vi "Get Message.vi"() -> (3 "message":string)   [LabVIEW 2014]
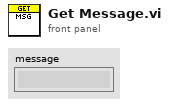
[diagram p1: front panel]
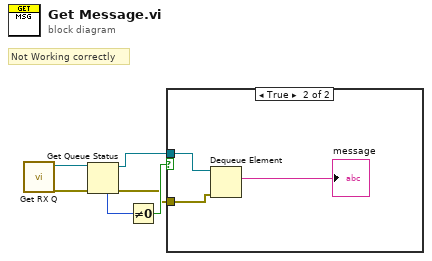
[diagram p0: block diagram]
diagram:
  # "Not Working correctly"
  n1 = call "Get RX Q.vi"() -> ("error out"=w5:errorcluster, "RX Q"=w6:refnum<queue>)  [unwired: 10 in]
  n2 = Get Queue Status(queue=w6, error in (no error)=w5) -> (queue out=w2:refnum<queue>, error out=w1:errorcluster, # elements in queue=w4:i32)  [unwired: 1 in, 5 out]
  n3 = Not Equal To 0?(x=w4) -> (x != 0?=w3:bool)
  n4 = case shown="True" w3 {
    tunnel: w2 -> [_ w8]
    tunnel: w1 -> [_ w7]
    frame False {
    }
    frame True {
      n5 = Dequeue Element(queue=w8, error in (no error)=w7) -> (element=→"message":string)  [unwired: 1 in, 3 out]
    }
  }
